vi "Pilot Analyze.vi"(5 "JoystickDevRef":T1) -> (2 "Suction":bool, 3 "x":dbl, 4 "y":dbl, 6 "Pull cables + telescope":bool, 8 "Release cable":bool, 10 "Transfer X control":bool, 15 "Slow Drive":bool)   [LabVIEW 2012]
uses:
  <vilib>/Rock Robotics/WPI/Joystick/WPI_JoystickDevRef.ctl
  <vilib>/Rock Robotics/WPI/Joystick/WPI_JoystickDeviceEnum.ctl
panel:
  out "Feeder":bool
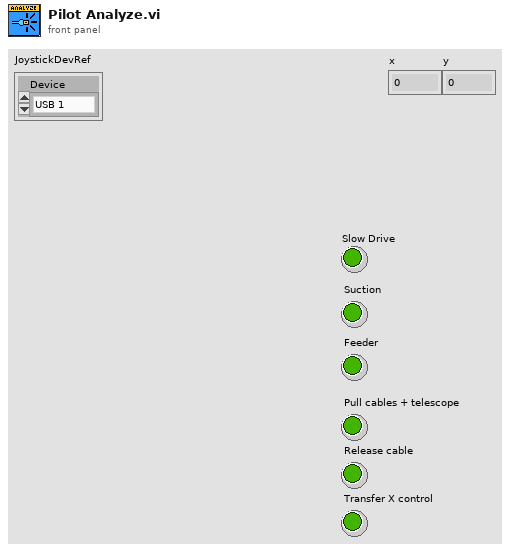
[diagram p1: front panel]
types:
  T1 = typedef "WPI_JoystickDevRef.ctl" = cluster{"Device":T2}
  T2 = typedef "WPI_JoystickDeviceEnum.ctl" = enum16{"USB 1", "USB 2", "USB 3", "USB 4", "Kinect 1", "Kinect 2"}
  T3 = typedef "WPI_JoystickButtonState.ctl" = cluster{"Button 1":bool, "Button 2":bool, "Button 3":bool, "Button 4":bool, "Button 5":bool, "Button 6":bool, "Button 7":bool, "Button 8":bool, "Button 9":bool, "Button 10":bool, "Button 11":bool, "Button 12":bool}
  T4 = cluster{"axis 1 (x)":dbl, "axis 2 (y)":dbl, "axis 3 (throttle)":dbl, "axis 4":dbl, "axis 5":dbl, "axis 6":dbl}
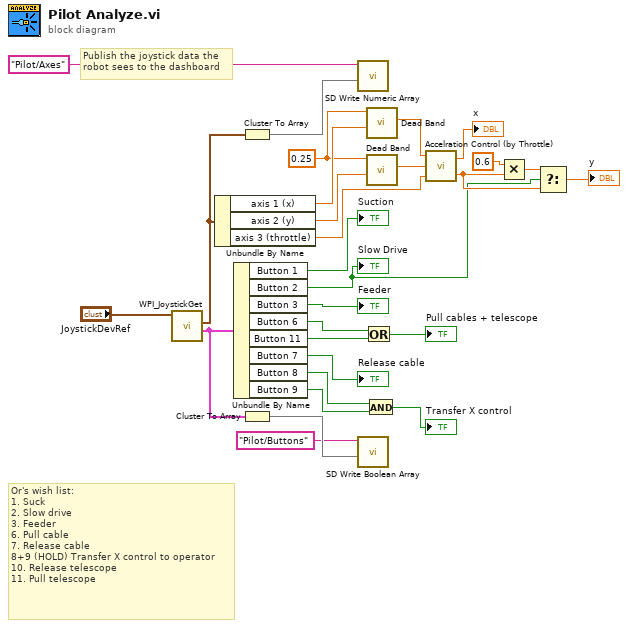
[diagram p0: block diagram]
diagram:
  w22 = 0.25 ("Dead Band")
  # "Or's wish list:\n1. Suck\n2. Slow drive\n3. Feeder\n6. Pull cable\n7. Release cable \n8+9 (HOLD) Transfer X control to operator\n10. Release telescope\n11. Pull telescope"
  # "Publish the joystick data the\nrobot sees to the dashboard"
  n1 = call <vilib>:"WPI_JoystickGet.vi"("JoystickDevRef"="JoystickDevRef") -> ("Buttons"=w14:T3, "Axes"=w15:T4)  [unwired: 4 in, 1 out]
  n2 = Unbundle By Name(w15) -> ("axis 1 (x)"=w26:dbl, "axis 2 (y)"=w24:dbl, "axis 3 (throttle)"=w13:dbl)
  n3 = Unbundle By Name(w14) -> ("Button 1"=→"Suction":bool, "Button 2"=w10:bool, "Button 3"=→"Feeder":bool, "Button 6"=w7:bool, "Button 11"=w6:bool, "Button 7"=→"Release cable":bool, "Button 8"=w2:bool, "Button 9"=w1:bool)
  "Slow Drive" <- w10
  n4 = Cluster To Array(cluster=w15) -> (array=w17:dbl[])
  n5 = Cluster To Array(cluster=w14) -> (array=w19:bool[])
  n6 = call <vilib>:"SD Write Numeric Array.vi"("Numeric Array"=w17, "Name"="Pilot/Axes") -> ()  [unwired: 8 in, 2 out]
  n7 = call <vilib>:"SD Write Boolean Array.vi"("Boolean Array"=w19, "Name"="Pilot/Buttons") -> ()  [unwired: 8 in, 2 out]
  n8 = Or(x=w7, y=w6) -> (x .or. y?=→"Pull cables + telescope":bool)
  n9 = And(x=w2, y=w1) -> (x .and. y?=→"Transfer X control":bool)
  n10 = call "Dead Band.vi"("Axis In"=w26, "Dead Band"=w22) -> ("Axis Out"=w25:dbl)  [unwired: 9 in]
  n11 = call "Dead Band.vi"("Axis In"=w24, "Dead Band"=w22) -> ("Axis Out"=w23:dbl)  [unwired: 9 in]
  n12 = call "Accelration Control (by Throttle).vi"("acc"=w13, "Yinput"=w23, "Xinput"=w25) -> ("Youtput"=w11:dbl, "Xoutput"=→"x":dbl)
  n13 = Multiply(x=0.6 ("y"), y=w11) -> (x*y=w21:dbl)
  n14 = Select(t=w21, s=w10, f=w11) -> (s? t:f=→"y":dbl)
